vi "testMain.vi"() -> ()   [LabVIEW 2014]
uses:
  Classes/Snake/Snake.lvclass
  TypeDefs/SnakeMovements.ctl
  <vilib>/Utility/inputDevices.llb/keyboardAcquire.vi
  <vilib>/Utility/inputDevices.llb/closeKeyboard.vi
panel:
  out "SnakeWorld":bool[][](array[boolean])
  out "Real 2D Array":u32[][](array[numeric])
  in  "stop":bool
  in  "StartPointX":i32=5
  in  "StartPointY":i32=5
  in  "FieldSizeY":i32=15
  in  "FieldSizeX":i32=10
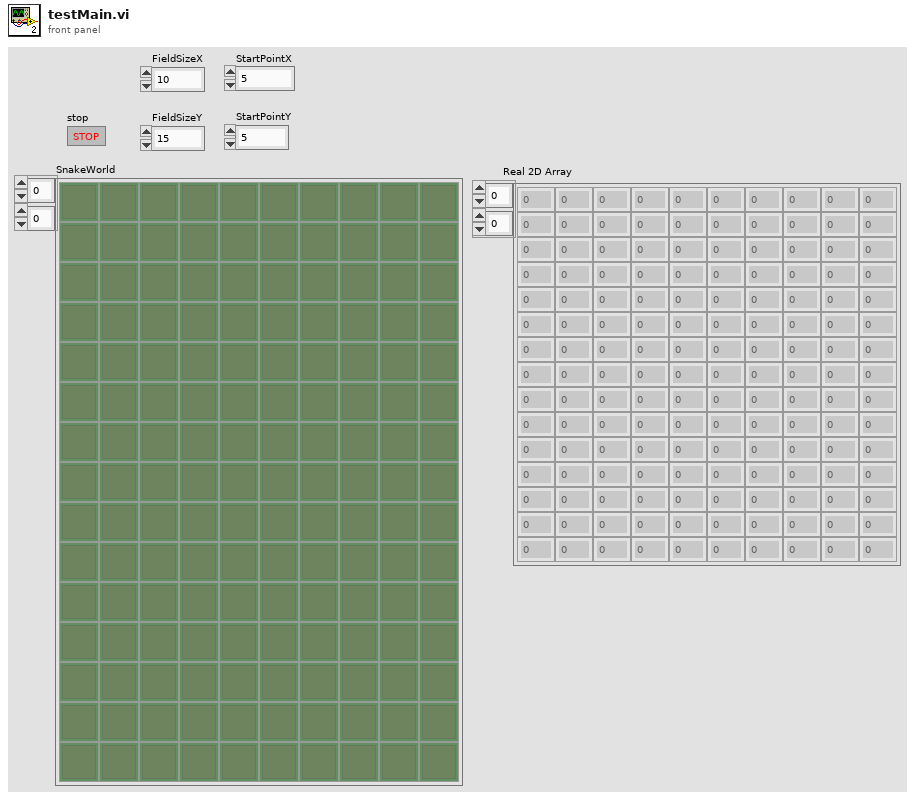
[diagram p1: front panel]
types:
  T1 = typedef "SnakeMovements.ctl" = enum16{"STOP", "UP", "DOWN", "RIGHT", "LEFT"}
  T2 = enum16{"0", "1", "2", "3", "4", "5", "6", "7", "8", "9", "A", "B", "C", "D", "E", "F", "G", "H", "I", "J", "K", "L", "M", "N", "O", "P", "Q", "R", "S", "T", "U", "V", "W", "X", "Y", "Z", "F1", "F2", "F3", "F4", "F5", "F6", "F7", "F8", "F9", "F10", "F11", "F12", "F13", "F14", "F15", "ADD", "BACK", "BACKSLASH", "CAPITAL", "COMMA", "DECIMAL", "DELETE", "DIVIDE", "DOWN", "END", "EQUALS", "ESCAPE", "GRAVE (`)", "HOME", "INSERT", "LBRACKET", "LCONTROL", "LEFT", "L ALT", "LSHIFT", "LWIN", "MINUS", "MULTIPLY", "NEXT", "NUMLOCK", "NUMPAD_0", "NUMPAD_1", "NUMPAD_2", "NUMPAD_3", "NUMPAD_4", "NUMPAD_5", "NUMPAD_6", "NUMPAD_7", "NUMPAD_8", "NUMPAD_9", "PAUSE", "PERIOD", "PRIOR (PG UP)", "RBRACKET", "RCONTROL", "RETURN", "RIGHT", "R ALT", "RSHIFT", "RWIN", "SCROLL", "SEMICOLON", "SLASH", "SPACE", "SUBTRACT", "TAB", "UP", "ENTER (num pad)", "' (quote)"}[]
  T3 = enum16{"0", "1", "2", "3", "4", "5", "6", "7", "8", "9", "A", "B", "C", "D", "E", "F", "G", "H", "I", "J", "K", "L", "M", "N", "O", "P", "Q", "R", "S", "T", "U", "V", "W", "X", "Y", "Z", "F1", "F2", "F3", "F4", "F5", "F6", "F7", "F8", "F9", "F10", "F11", "F12", "F13", "F14", "F15", "ADD", "BACK", "BACKSLASH", "CAPITAL", "COMMA", "DECIMAL", "DELETE", "DIVIDE", "DOWN", "END", "EQUALS", "ESCAPE", "GRAVE (`)", "HOME", "INSERT", "LBRACKET", "LCONTROL", "LEFT", "L ALT", "LSHIFT", "LWIN", "MINUS", "MULTIPLY", "NEXT", "NUMLOCK", "NUMPAD_0", "NUMPAD_1", "NUMPAD_2", "NUMPAD_3", "NUMPAD_4", "NUMPAD_5", "NUMPAD_6", "NUMPAD_7", "NUMPAD_8", "NUMPAD_9", "PAUSE", "PERIOD", "PRIOR (PG UP)", "RBRACKET", "RCONTROL", "RETURN", "RIGHT", "R ALT", "RSHIFT", "RWIN", "SCROLL", "SEMICOLON", "SLASH", "SPACE", "SUBTRACT", "TAB", "UP", "ENTER (num pad)", "' (quote)"}
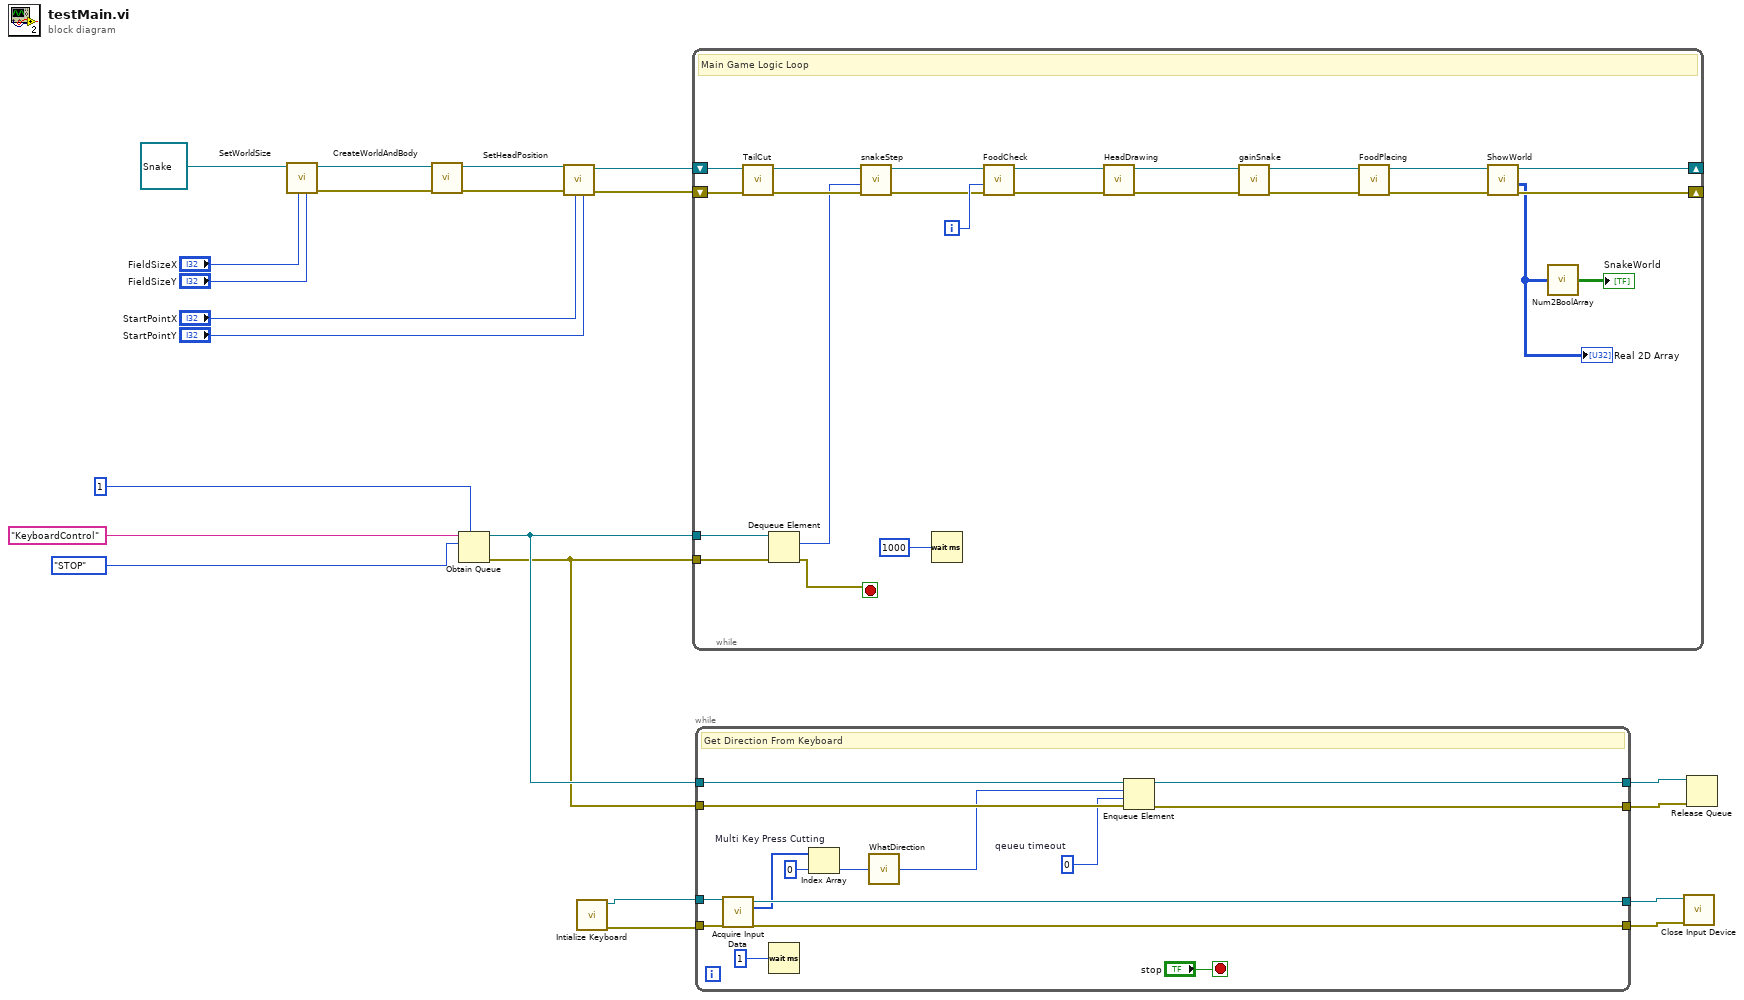
[diagram p0: block diagram]
diagram:
  n1 = call-dynamic "SetWorldSize.vi"("WorldSizeY"="FieldSizeY", "WorldSizeX"="FieldSizeX", "Snake in"=refnum<class "Snake.lvclass"> refnum ("Snake.lvclass")) -> ("error out"=w13:errorcluster, "Snake out"=w14:refnum<class "Snake.lvclass">)  [unwired: 7 in]
  n2 = call-dynamic "CreateWorldAndBody.vi"("error in (no error)"=w13, "Snake in"=w14) -> ("error out"=w21:errorcluster, "Snake out"=w22:refnum<class "Snake.lvclass">)  [unwired: 8 in]
  n3 = Obtain Queue(max queue size (-1, unlimited)=1, name (unnamed)="KeyboardControl", element data type=SnakeMovements."STOP" ("Movement")) -> (queue out=w8:refnum<queue>, error out=w7:errorcluster)  [unwired: 2 in, 1 out]
  n4 = call-dynamic "SetHeadPosition.vi"("HeadPositionY"="StartPointY", "HeadPositionX"="StartPointX", "error in (no error)"=w21, "Snake in"=w22) -> ("error out"=w9:errorcluster, "Snake out"=w10:refnum<class "Snake.lvclass">)  [unwired: 6 in]
  n5 = call <vilib>:"Intialize Keyboard.vi"() -> ("error out"=w5:errorcluster, "device ID"=w6:refnum<k1>)  [unwired: 10 in]
  n6 = while {
    tunnel: w8 -> [w46]
    tunnel: w7 -> [w37]
    shift-right: [w31] -> _
    shift-left: w10 -> [w45]
    shift-right: [w32] -> _
    shift-left: w9 -> [w44]
    i -> [w38]
    stop <- w29 stop-if-true
    # "Main Game Logic Loop"
    n7 = call-dynamic "TailCut.vi"("error in (no error)"=w44, "Snake in"=w45) -> ("error out"=w42:errorcluster, "Snake out"=w43:refnum<class "Snake.lvclass">)  [unwired: 8 in]
    n8 = Dequeue Element(queue=w46, error in (no error)=w37) -> (element=w41:T1, error out=w29:errorcluster)  [unwired: 1 in, 2 out]
    n9 = call-dynamic "snakeStep.vi"("error in (no error)"=w42, "Movement"=w41, "Snake in"=w43) -> ("error out"=w27:errorcluster, "Snake out"=w28:refnum<class "Snake.lvclass">)  [unwired: 7 in]
    n10 = Wait (ms)(milliseconds to wait=u32 1000) -> ()  [unwired: 1 out]
    n11 = call-dynamic "FoodCheck.vi"("error in (no error)"=w27, "IterationNumber"=w38, "Snake in"=w28) -> ("error out"=w25:errorcluster, "Snake out"=w26:refnum<class "Snake.lvclass">)  [unwired: 7 in]
    n12 = call-dynamic "HeadDrawing.vi"("error in (no error)"=w25, "Snake in"=w26) -> ("error out"=w23:errorcluster, "Snake out"=w24:refnum<class "Snake.lvclass">)  [unwired: 8 in]
    n13 = call-dynamic "gainSnake.vi"("error in (no error)"=w23, "Snake in"=w24) -> ("error out"=w39:errorcluster, "Snake out"=w40:refnum<class "Snake.lvclass">)  [unwired: 8 in]
    n14 = call-dynamic "FoodPlacing.vi"("error in (no error)"=w39, "Snake in"=w40) -> ("error out"=w33:errorcluster, "Snake out"=w34:refnum<class "Snake.lvclass">)  [unwired: 8 in]
    n15 = call-dynamic "ShowWorld.vi"("error in (no error)"=w33, "Snake in"=w34) -> ("error out"=w32:errorcluster, "SnakeWorldAndBody"=w30:u32[][], "Snake out"=w31:refnum<class "Snake.lvclass">)  [unwired: 7 in]
    "Real 2D Array" <- w30
    n16 = call "Num2BoolArray.vi"("Real 2D Array"=w30) -> ("BooleanArray"=→"SnakeWorld":bool[][])
  }
  n17 = while {
    tunnel: w6 -> [w61]
    tunnel: w5 -> [w60]
    tunnel: [w59] -> w2
    tunnel: [w58] -> w1
    tunnel: w7 -> [w52]
    tunnel: w8 -> [w53]
    tunnel: [w50] -> w4
    tunnel: [w49] -> w3
    stop <- "stop" stop-if-true
    w48 = 0  # qeueu timeout
    # "Get Direction From Keyboard"
    n18 = call-poly <vilib>:"Acquire Input Data.vi"("device ID"=w61, "error in (no error)"=w60) -> ("device ID"=w59:refnum<k1>, "keys pressed"=w56:T2, "error out"=w58:errorcluster)  [unwired: 15 in]
    n19 = Wait (ms)(milliseconds to wait=u32 1) -> ()  [unwired: 1 out]
    n20 = Index Array "Multi Key Press Cutting"(array=w56, index=0) -> (element=w54:T3)
    n21 = call "WhatDirection.vi"("key"=w54) -> ("Movement"=w51:T1)
    n22 = Enqueue Element(queue=w53, element=w51, timeout in ms (-1)=w48, error in (no error)=w52) -> (queue out=w50:refnum<queue>, error out=w49:errorcluster)  [unwired: 1 out]
  }
  n23 = call-poly <vilib>:"Close Input Device.vi"("error in (no error)"=w1, "device ID"=w2) -> ()  [unwired: 8 in, 1 out]
  n24 = Release Queue(queue=w4, error in (no error)=w3) -> ()  [unwired: 1 in, 3 out]
